vi "_Check Model Family.vi"(1 "Model Family (100)":T1=1 items=["8080 Series", "100 Series", "200 Series", "300 Series", "Other Series"]) -> (0 "Yes":bool)   [LabVIEW 2015]
uses:
  Type/_Model Family.ctl
  Type/_Instrument Model.ctl
  Configuration/_Global Configuration.vi
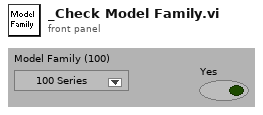
[diagram p1: front panel]
types:
  T1 = typedef "_Model Family.ctl" = u16
  T2 = typedef "_Instrument Model.ctl" = enum16{"QSight 110", "QSight 120", "QSight 210", "QSight 220", "QSight 410", "QSight 420", "IONICS 3Q 110", "IONICS 3Q 120", "IONICS 3Q 210", "IONICS 3Q 220", "IONICS 3Q 310", "IONICS 3Q 320", "Simulation (Single Source)", "Simulation (Dual Source)"}
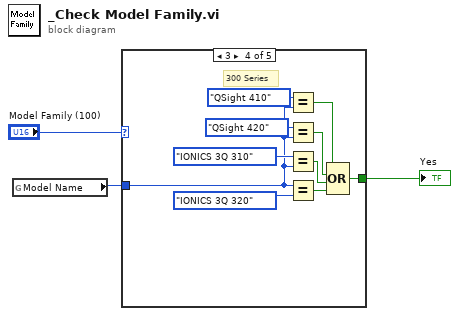
[diagram p0: block diagram]
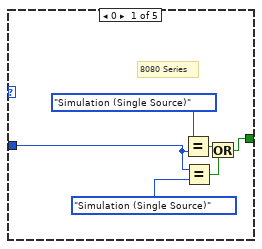
[diagram p2: hidden frame]
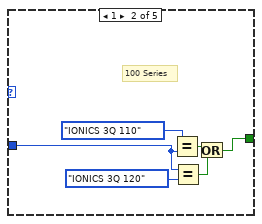
[diagram p3: hidden frame]
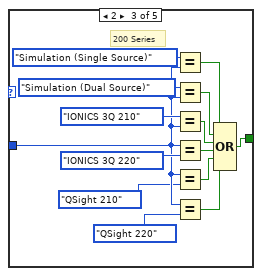
[diagram p4: hidden frame]
diagram:
  n1 = global read "_Global Configuration.vi" "Model Name"() -> (w2:T2)
  n2 = case shown="3" "Model Family (100)" {
    tunnel: [w4 w15 w29 w39 _] -> w3
    tunnel: w2 -> [w5 w10 w18 w30 _]
    frame 0 {
      # "8080 Series"
      n3 = Equal?(x=_Instrument_Model."Simulation (Single Source)" ("y"), y=w5) -> (x = y?=w8:bool)
      n4 = Equal?(x=w5, y=_Instrument_Model."Simulation (Single Source)") -> (x = y?=w9:bool)
      n5 = Or(x=w8, y=w9) -> (x .or. y?=w4:bool)
    }
    frame 1 {
      # "100 Series"
      n6 = Equal?(x=_Instrument_Model."IONICS 3Q 110" ("y"), y=w10) -> (x = y?=w13:bool)
      n7 = Equal?(x=w10, y=_Instrument_Model."IONICS 3Q 120") -> (x = y?=w14:bool)
      n8 = Or(x=w13, y=w14) -> (x .or. y?=w15:bool)
    }
    frame 2 {
      # "200 Series"
      n9 = Equal?(x=_Instrument_Model."Simulation (Single Source)" ("y"), y=w18) -> (x = y?=w19:bool)
      n10 = Equal?(x=_Instrument_Model."Simulation (Dual Source)" ("y"), y=w18) -> (x = y?=w20:bool)
      n11 = Equal?(x=_Instrument_Model."IONICS 3Q 210" ("y"), y=w18) -> (x = y?=w26:bool)
      n12 = Equal?(x=w18, y=_Instrument_Model."IONICS 3Q 220") -> (x = y?=w24:bool)
      n13 = Equal?(x=w18, y=_Instrument_Model."QSight 210") -> (x = y?=w23:bool)
      n14 = Equal?(x=w18, y=_Instrument_Model."QSight 220") -> (x = y?=w25:bool)
      n15 = Compound Arithmetic op=OR(w19, w20, w26, w24, w23, w25) -> (w29:bool)
    }
    frame 3 {
      # "300 Series"
      n16 = Equal?(x=_Instrument_Model."QSight 410" ("y"), y=w30) -> (x = y?=w31:bool)
      n17 = Equal?(x=_Instrument_Model."QSight 420" ("y"), y=w30) -> (x = y?=w32:bool)
      n18 = Equal?(x=_Instrument_Model."IONICS 3Q 310" ("y"), y=w30) -> (x = y?=w36:bool)
      n19 = Equal?(x=w30, y=_Instrument_Model."IONICS 3Q 320") -> (x = y?=w35:bool)
      n20 = Compound Arithmetic op=OR(w31, w32, w36, w35) -> (w39:bool)
    }
    frame Default {
    }
  }
  "Yes" <- w3
